vi "5-1-2 delay imposto no error.vi"(1 "error in":bool, 2 "delay":u32=500) -> (0 "error out":bool)   [LabVIEW 2012]
doc: "© Copyright M. Ferrari 2000\n Delay function"
panel:
  # "Realizzare un VI che permetta di impostare un certo ritardo, in ms, attraverso l'ingresso 'delay' e di \ntrasferire il valore di 'error in' all'uscita 'error out'. Se  presente un errore in ingresso non dovr essere\ngenerato alcun ritardo."
  # "[ms]"
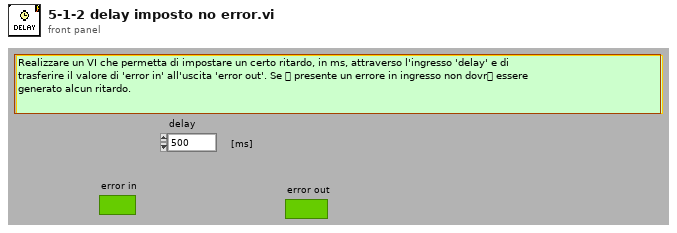
[diagram p1: front panel]
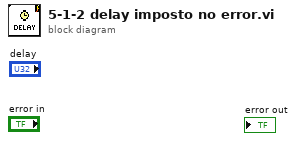
[diagram p0: block diagram]
diagram:
